vi "19_DC Motor_PID_final.vi"() -> ()   [LabVIEW 2018]
uses:
  <userlib>/KNR OS 4.0 LabVIEW Toolkit/Type Definition/Resource.ctl
  <userlib>/KNR OS 4.0 LabVIEW Toolkit/Type Definition/DC Motor Port.ctl
panel:
  in  "Reset 2":bool
  in  "Reverse? 2":bool
  out "Velocity (cm/sec) 2":dbl
  out "Position cm 2":dbl
  out "Speed (+-100%) 2":dbl
  out "Speed (+-100%)":dbl
  in  "Desire Velosity (cm/sec)":dbl(slide) scale=-200.0..200.0
  in  "IP":string(combo)="172.22.11.2"
  in  "Resource":T1=enum."KNRm_DDDD"
  in  "stop":bool
  in  "Enable Motor":bool
  out "Position cm":dbl
  out "Velocity (cm/sec)":dbl
  in  "Reverse?":bool
  in  "Reset":bool
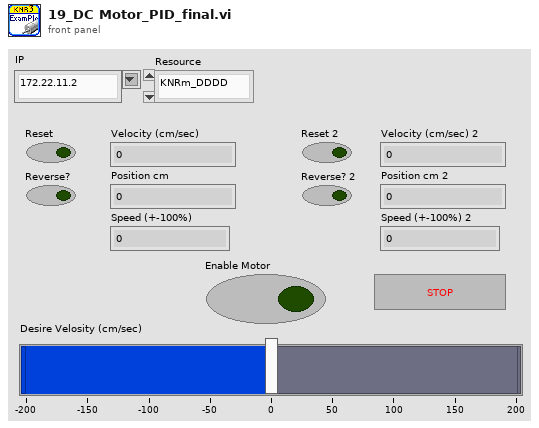
[diagram p1: front panel]
types:
  T1 = typedef "Resource.ctl" = enum16{"KNRm_DDRC", "KNRm_DDDD", "KNRm_DDDR", "KNRm_DDDC", "KNR", "KNRm_neww"}
  T2 = typedef "KNR3 Reference.ctl" = cluster{"FPGA Session":refnum<class "FPGA Interface Base.lvclass">, "Resource":T1}
  T3 = typedef "DC Motor Port.ctl" = u16
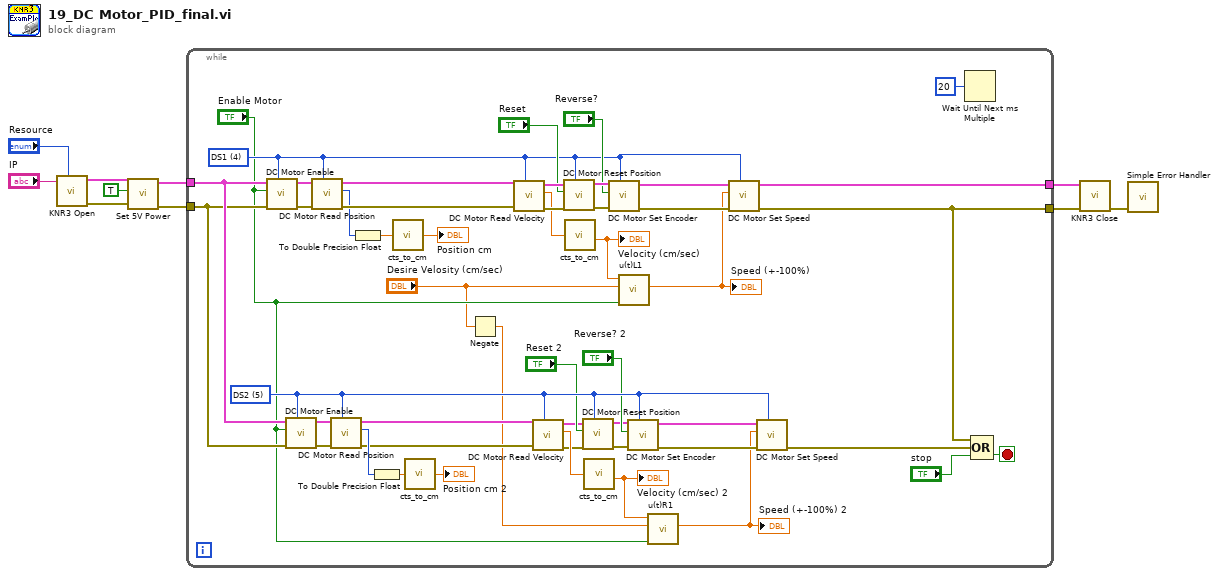
[diagram p0: block diagram]
diagram:
  n1 = call <userlib>:"KNR3 Open.vi"("Resource"="Resource", "IP"="IP") -> ("error out"=w4:errorcluster, "KNR out"=w6:T2)  [unwired: 8 in]
  n2 = call <userlib>:"Set 5V Power.vi"("error in (no error)"=w4, "5V Power(T)"=TRUE ("5V Power"), "KNR in"=w6) -> ("error out"=w8:errorcluster, "KNR out"=w9:T2)  [unwired: 7 in]
  n3 = while {
    tunnel: w9 -> [w19]
    tunnel: w8 -> [w18]
    tunnel: [w39] -> w2
    tunnel: [w17] -> w1
    stop <- w58 stop-if-true
    w36 = T3 5 items=["DS1"=4, "DS2"=5, "DS3"=6, "DS4"=7] ("Port 2")
    w40 = T3 4 items=["DS1"=4, "DS2"=5, "DS3"=6, "DS4"=7] ("Port")
    n4 = call <userlib>:"DC Motor Enable.vi"("Port (DS1)"=w40, "error in (no error)"=w18, "Enable Motor(F)"="Enable Motor", "KNR in"=w19) -> ("error out"=w43:errorcluster, "KNR out"=w44:T2)  [unwired: 6 in]
    n5 = call <userlib>:"DC Motor Enable.vi"("Port (DS1)"=w36, "error in (no error)"=w18, "Enable Motor(F)"="Enable Motor", "KNR in"=w19) -> ("error out"=w33:errorcluster, "KNR out"=w32:T2)  [unwired: 6 in]
    n6 = call <userlib>:"DC Motor Read Position.vi"("Port (DS1)"=w40, "error in (no error)"=w43, "KNR in"=w44) -> ("error out"=w55:errorcluster, "Position"=w46:i32, "KNR out"=w56:T2)  [unwired: 6 in]
    n7 = call <userlib>:"DC Motor Read Position.vi"("Port (DS1)"=w36, "error in (no error)"=w33, "KNR in"=w32) -> ("error out"=w21:errorcluster, "Position"=w30:i32, "KNR out"=w20:T2)  [unwired: 6 in]
    n8 = To Double Precision Float(number=w46) -> (double precision float=w45:dbl)
    n9 = To Double Precision Float(number=w30) -> (double precision float=w31:dbl)
    n10 = call "cts_to_cm.vi"("cts"=w45) -> ("cm"=→"Position cm":dbl)
    n11 = call "cts_to_cm.vi"("cts"=w31) -> ("cm"=→"Position cm 2":dbl)
    n12 = Negate(x="Desire Velosity (cm/sec)") -> (-x=w12:dbl)
    n13 = call <userlib>:"DC Motor Read Velocity.vi"("Port (DS1)"=w40, "error in (no error)"=w55, "KNR in"=w56) -> ("error out"=w51:errorcluster, "Velocity (cts/sec)"=w50:dbl, "KNR out"=w54:T2)  [unwired: 6 in]
    n14 = call <userlib>:"DC Motor Read Velocity.vi"("Port (DS1)"=w36, "error in (no error)"=w21, "KNR in"=w20) -> ("error out"=w25:errorcluster, "Velocity (cts/sec)"=w26:dbl, "KNR out"=w22:T2)  [unwired: 6 in]
    n15 = call <userlib>:"DC Motor Reset Position.vi"("Port (DS1)"=w40, "error in (no error)"=w51, "Reset(F)"="Reset", "KNR in"=w54) -> ("error out"=w52:errorcluster, "KNR out"=w53:T2)  [unwired: 6 in]
    n16 = call "cts_to_cm.vi"("cts"=w50) -> ("cm"=w38:dbl)
    "Velocity (cm/sec)" <- w38
    n17 = call <userlib>:"DC Motor Reset Position.vi"("Port (DS1)"=w36, "error in (no error)"=w25, "Reset(F)"="Reset 2", "KNR in"=w22) -> ("error out"=w24:errorcluster, "KNR out"=w23:T2)  [unwired: 6 in]
    n18 = call "cts_to_cm.vi"("cts"=w26) -> ("cm"=w15:dbl)
    "Velocity (cm/sec) 2" <- w15
    n19 = call <userlib>:"DC Motor Set Encoder.vi"("Port (DS1)"=w40, "error in (no error)"=w52, "Reverse?(F)"="Reverse?", "KNR in"=w53) -> ("error out"=w41:errorcluster, "KNR out"=w42:T2)  [unwired: 6 in]
    n20 = call "u(t)L1.vi"("Velocity"=w38, "Desire Velosity"="Desire Velosity (cm/sec)", "enable"="Enable Motor") -> ("u(t)"=w37:dbl)  [unwired: 7 in]
    "Speed (+-100%)" <- w37
    n21 = call <userlib>:"DC Motor Set Encoder.vi"("Port (DS1)"=w36, "error in (no error)"=w24, "Reverse?(F)"="Reverse? 2", "KNR in"=w23) -> ("error out"=w35:errorcluster, "KNR out"=w34:T2)  [unwired: 6 in]
    n22 = call "u(t)R1.vi"("Velocity"=w15, "Desire Velosity"=w12, "enable"="Enable Motor") -> ("u(t)"=w13:dbl)  [unwired: 7 in]
    "Speed (+-100%) 2" <- w13
    n23 = call <userlib>:"DC Motor Set Speed.vi"("Port (DS1)"=w40, "error in (no error)"=w41, "Speed (+-100%)"=w37, "KNR in"=w42) -> ("error out"=w17:errorcluster, "KNR out"=w39:T2)  [unwired: 6 in]
    n24 = call <userlib>:"DC Motor Set Speed.vi"("Port (DS1)"=w36, "error in (no error)"=w35, "Speed (+-100%)"=w13, "KNR in"=w34) -> ("error out"=w16:errorcluster)  [unwired: 6 in, 1 out]
    n25 = Wait Until Next ms Multiple(millisecond multiple=u32 20) -> ()  [unwired: 1 out]
    n26 = Compound Arithmetic op=OR(w17, w16, "stop") -> (w58:bool)
  }
  n27 = call <userlib>:"KNR3 Close.vi"("error in (no error)"=w1, "KNR in"=w2) -> ("error out"=w7:errorcluster)  [unwired: 9 in]
  n28 = call <vilib>:"Simple Error Handler.vi"("error in (no error)"=w7) -> ()  [unwired: 4 in, 5 out]
